vi "Save String to Control.vi"(10 "value":string, 11 "Control":refnum<vi>) -> ()   [LabVIEW 2014]
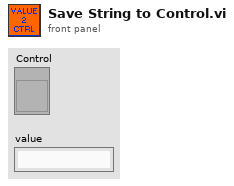
[diagram p1: front panel]
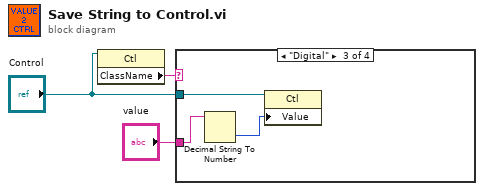
[diagram p0: block diagram]
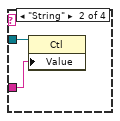
[diagram p3: hidden frame]
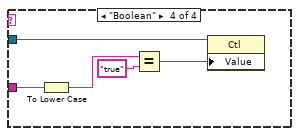
[diagram p4: hidden frame]
diagram:
  n1 = property class="Ctl"(reference="Control") -> ("ClassName"=w1:string)  [unwired: 1 in, 2 out]
  n2 = case shown="\"Digital\"" w1 {
    tunnel: "Control" -> [_ w5 w8 w13]
    tunnel: "value" -> [_ w4 w7 w12]
    frame "False", Default {
      # "Do something here to \ncatch errors and add \ncases to handle various\nclasses"
    }
    frame "String" {
      n3 = property class="Ctl"(reference=w5, "Value"=w4) -> ()  [unwired: 1 in, 2 out]
    }
    frame "Digital" {
      n4 = Decimal String To Number(string=w7) -> (number=w6:i32)  [unwired: 2 in, 1 out]
      n5 = property class="Ctl"(reference=w8, "Value"=w6) -> ()  [unwired: 1 in, 2 out]
    }
    frame "Boolean" {
      n6 = To Lower Case(string=w12) -> (all lower case string=w11:string)
      n7 = Equal?(x=w11, y="true") -> (x = y?=w9:bool)
      n8 = property class="Ctl"(reference=w13, "Value"=w9) -> ()  [unwired: 1 in, 2 out]
    }
  }
